vi "FGV AK Befehl aktiv.vi"(6 "Aktion":enum16{"initialisieren", "lesen", "schreiben"}(ring), 11 "Cluster (in)":cluster{"Befehl von AK":bool}) -> (3 "Cluster (out)":cluster{"Befehl von AK":bool})   [LabVIEW 2015, in "AK-Schnittstelle.lvlib"]
uses:
  AK-Schnittstelle.lvlib
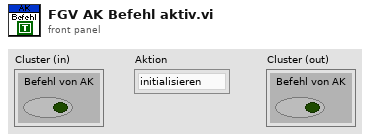
[diagram p1: front panel]
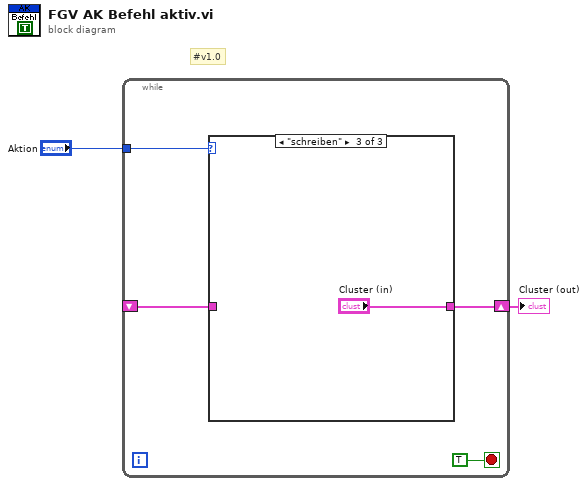
[diagram p0: block diagram]
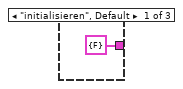
[diagram p2: hidden frame]
diagram:
  # "#v1.0"
  n1 = while {
    tunnel: "Aktion" -> [w5]
    shift-right: [w4] -> w1
    shift-left: _ -> [w3]
    stop <- TRUE stop-if-true
    n2 = case shown="\"schreiben\"" w5 {
      tunnel: [cluster{"Befehl von AK":bool} {"Befehl von AK"=FALSE} ("Cluster (in)") w8 "Cluster (in)"] -> w4
      tunnel: w3 -> [_ w8 _]
      frame "initialisieren", Default {
      }
      frame "lesen" {
      }
      frame "schreiben" {
      }
    }
  }
  "Cluster (out)" <- w1
